vi "MathUtil_RateOfChange.vi"(6 "FPGA_Time_Seconds":dbl=-1.0, 11 "Input":dbl) -> (3 "Rate_Of_Change":dbl)   [LabVIEW 2019, in "Trajectory_Library.lvlib"]
doc: "Calculate the rate of change (Units/Second) of an input value (Units).\n\nInputs:\n - Input - double - Value to calculate rate of change for.\n - FPGA Time - double - FPGA time stamp (optional).\n\nOutputs:\n - RateOfChange - double - Calculated rate of change of input value."
uses:
  Trajectory_Library.lvlib
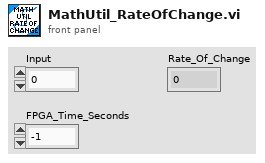
[diagram p1: front panel]
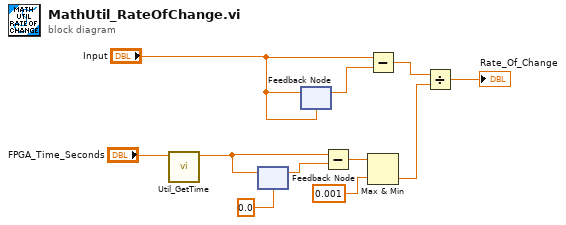
[diagram p0: block diagram]
diagram:
  n1 = call "Util_GetTime.vi"("Pass_Through_Time"="FPGA_Time_Seconds") -> ("FPGA_Time_Seconds"=w1:dbl)  [unwired: 8 in, 2 out]
  n2 = feedback #1(0.0 ("FPGA_Time_Seconds")) -> (w9:dbl)
  n3 = feedback-in #1(w1) -> ()
  n4 = feedback #2("Input") -> (w8:dbl)
  n5 = feedback-in #2("Input") -> ()
  n6 = Subtract(x=w1, y=w9) -> (x-y=w3:dbl)
  n7 = Subtract(x="Input", y=w8) -> (x-y=w5:dbl)
  n8 = Max & Min(x=w3, y=0.001) -> (min(x,y)=w6:dbl)  [unwired: 1 out]
  n9 = Divide(x=w5, y=w6) -> (x/y=→"Rate_Of_Change":dbl)
